vi "S2C_VLFT10_Proc_Globals.vi"() -> ()   [LabVIEW 2015]
doc: "Globals for the 5190CR process."
panel:
  out "VLFT10-Tcp":refnum<k5>
  out "VLFT10-Refs":string[][](array[string])
  in  "VLFT10-VI":refnum<vi>
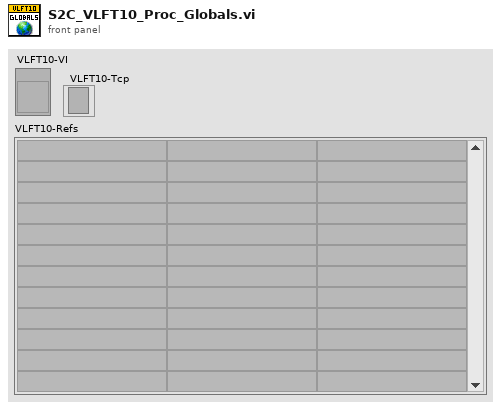
[diagram p1: front panel]
diagram:
